vi "YPRGlobal.vi"(0 "Yaw":dbl, 1 "Pitch":dbl, 2 "Roll":dbl, 3 "Compass Heading":dbl, 7 "Byte Count":u32, 8 "Update":bool, 10 "Initialize":bool) -> (20 "Yaw Out":dbl, 21 "Pitch Out":dbl, 22 "Roll Out":dbl, 23 "Compass Heading Out":dbl, 25 "Last Update":dbl, 26 "Update Count":i32, 27 "Byte Count Out":u32)   [LabVIEW 2013, in "Nav6.lvlib"]
uses:
  Nav6.lvlib
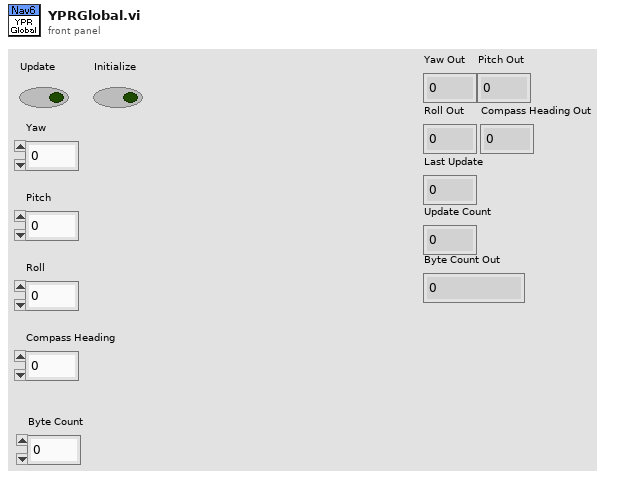
[diagram p1: front panel]
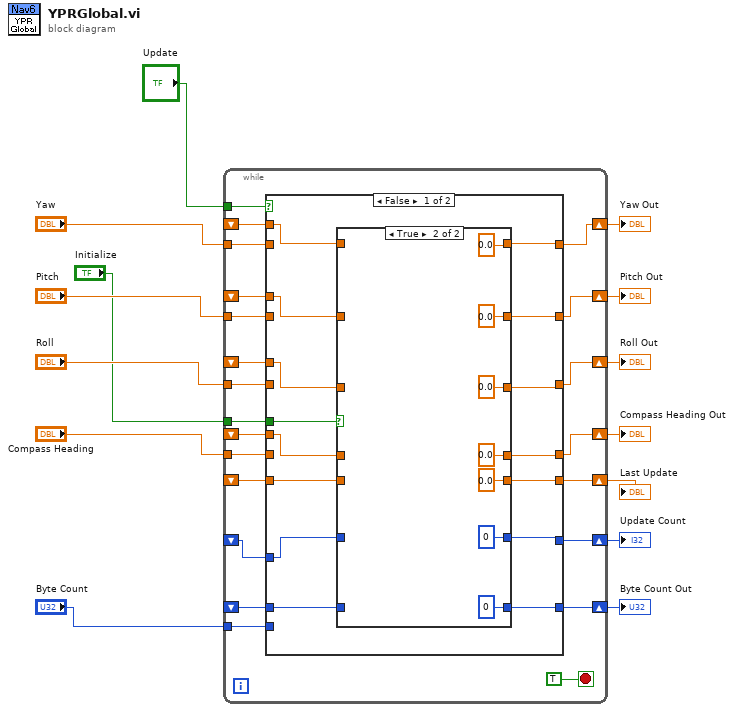
[diagram p0: block diagram]
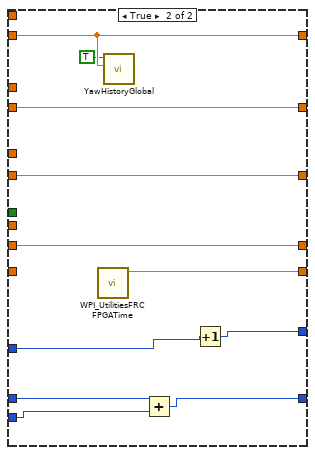
[diagram p3: hidden frame]
diagram:
  n1 = while {
    shift-right: [w34] -> w10
    shift-left: _ -> [w27]
    shift-right: [w32] -> w9
    shift-left: _ -> [w26]
    shift-right: [w30] -> w8
    shift-left: _ -> [w25]
    shift-right: [w28] -> w7
    shift-left: _ -> [w24]
    tunnel: "Yaw" -> [w35]
    tunnel: "Pitch" -> [w33]
    tunnel: "Roll" -> [w31]
    tunnel: "Compass Heading" -> [w29]
    shift-right: [w23] -> w6
    shift-left: _ -> [w22]
    shift-right: [w21] -> w4
    shift-left: _ -> [w20]
    shift-right: [w18] -> w3
    shift-left: _ -> [w19]
    tunnel: "Byte Count" -> [w17]
    tunnel: "Update" -> [w16]
    tunnel: "Initialize" -> [w15]
    stop <- TRUE stop-if-true
    n2 = case shown="False" w16 {
      tunnel: [w50 w72] -> w34
      tunnel: w35 -> [_ w72]
      tunnel: [w48 w76] -> w32
      tunnel: w33 -> [_ w76]
      tunnel: [w46 w75] -> w30
      tunnel: w31 -> [_ w75]
      tunnel: [w44 w74] -> w28
      tunnel: w29 -> [_ w74]
      tunnel: w27 -> [w51 _]
      tunnel: w26 -> [w49 _]
      tunnel: w25 -> [w47 _]
      tunnel: w24 -> [w45 _]
      tunnel: [w42 w73] -> w23
      tunnel: w22 -> [w43 _]
      tunnel: [w40 w67] -> w21
      tunnel: w20 -> [w41 w66]
      tunnel: [w38 w68] -> w18
      tunnel: w19 -> [w39 w69]
      tunnel: w17 -> [_ w70]
      tunnel: w15 -> [w37 _]
      frame False {
        n3 = case shown="True" w37 {
          tunnel: w51 -> [w58 _]
          tunnel: [w58 0.0 ("Yaw")] -> w50
          tunnel: w49 -> [w57 _]
          tunnel: [w57 0.0 ("Pitch")] -> w48
          tunnel: w47 -> [w56 _]
          tunnel: [w56 0.0 ("Roll")] -> w46
          tunnel: w45 -> [w55 _]
          tunnel: [w55 0.0 ("Compass Heading")] -> w44
          tunnel: w43 -> [w54 _]
          tunnel: [w54 0.0 ("FPGA Time")] -> w42
          tunnel: w41 -> [w53 _]
          tunnel: [w53 u32 0] -> w40
          tunnel: w39 -> [w52 _]
          tunnel: [w52 u32 0] -> w38
          frame False {
          }
          frame True {
          }
        }
      }
      frame True {
        n4 = call <vilib>:"WPI_UtilitiesFRC FPGATime.vi"() -> ("FPGA Time"=w73:dbl)  [unwired: 10 in, 1 out]
        n5 = call "YawHistoryGlobal.vi"("Yaw"=w72, "Update"=TRUE) -> ()  [unwired: 9 in, 1 out]
        n6 = Add(x=w69, y=w70) -> (x+y=w68:u32)
        n7 = Increment(x=w66) -> (x+1=w67:u32)
      }
    }
  }
  "Yaw Out" <- w10
  "Pitch Out" <- w9
  "Roll Out" <- w8
  "Compass Heading Out" <- w7
  "Last Update" <- w6
  "Update Count" <- w4
  "Byte Count Out" <- w3
